vi "Write WaveformFactory.vi"(10 "WaveformFactory":refnum<class "IWaveformFactory.lvclass">, 11 "Model in":refnum<class "Model.lvclass">) -> (3 "Model out":refnum<class "Model.lvclass">)   [LabVIEW 2015, in "Model.lvclass"]
uses:
  Model.lvclass
  WaveformFactory/IWaveformFactory/IWaveformFactory.lvclass
  Model.lvclass/Model.ctl
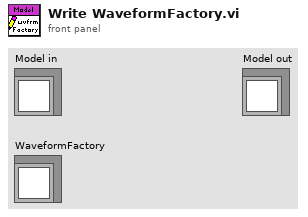
[diagram p1: front panel]
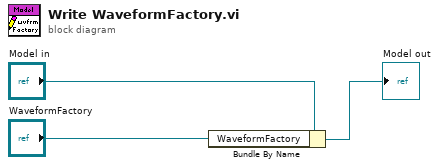
[diagram p0: block diagram]
diagram:
  n1 = Bundle By Name(cluster="Model in", "WaveformFactory"="WaveformFactory") -> (→"Model out":refnum<class "Model.lvclass">)
